vi "image read.vi"() -> ()   [LabVIEW 2021]
panel:
  out "error out 2":errorcluster
  out "error out":errorcluster
  out "Image":T1(plugin-control)
  in  "File Path":path
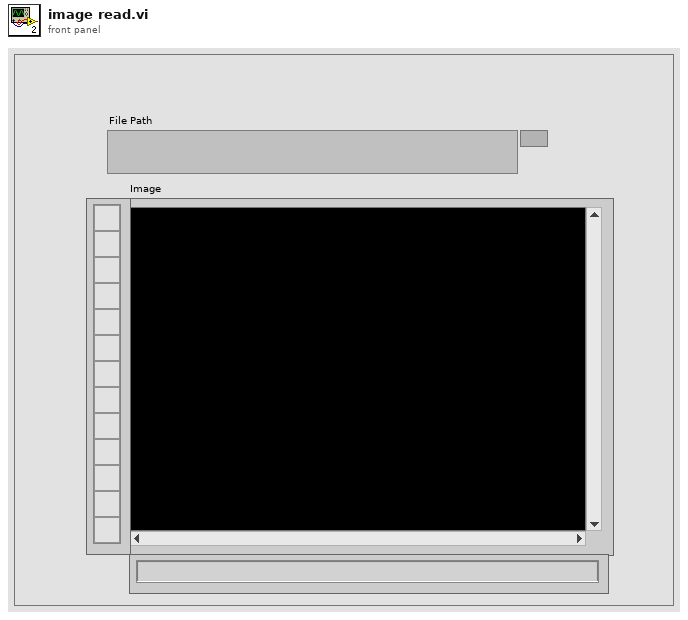
[diagram p1: front panel]
types:
  T1 = typedef "IMAQ Image.ctl" = refnum<image>
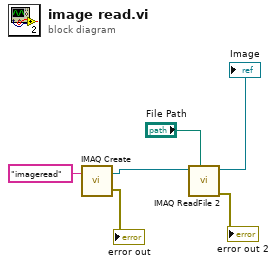
[diagram p0: block diagram]
diagram:
  n1 = call "IMAQ Create"("Image Name"="imageread") -> ("New Image"=w4:T1, "error out"=→"error out":errorcluster)  [unwired: 4 in]
  n2 = call "IMAQ ReadFile 2"("File Path"="File Path", "Image"=w4) -> ("error out"=→"error out 2":errorcluster, "Image Out"=→"Image":T1)  [unwired: 5 in, 3 out]
